vi "SyncMatrixGen (SubVI).vi"(9 "M":i32, 10 "Hamming distance":i32, 11 "Length":i32) -> (3 "Array":i32[][](array[numeric]))   [LabVIEW 2017]
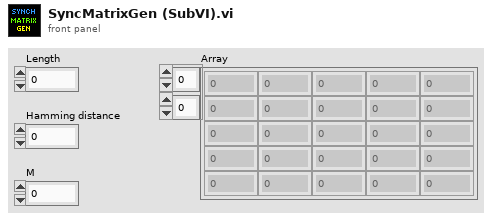
[diagram p1: front panel]
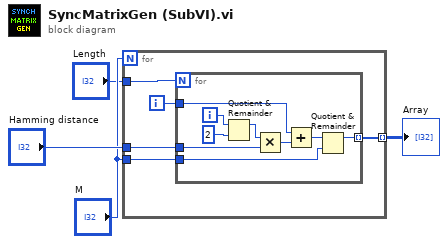
[diagram p0: block diagram]
diagram:
  n1 = for {
    N: "M" -> [_]
    tunnel: "Length" -> [w9]
    tunnel: [w8] -> w2 mode=indexing
    tunnel: "M" -> [w6]
    tunnel: "Hamming distance" -> [w5]
    i -> [w7]
    n2 = for {
      N: w9 -> [_]
      tunnel: [w12] -> w8 mode=indexing
      tunnel: w7 -> [w14]
      tunnel: w6 -> [w11]
      tunnel: w5 -> [w10]
      i -> [w18]
      n3 = Quotient & Remainder(x=w18, y=2) -> (x-y*floor(x/y)=w16:i32)  [unwired: 1 out]
      n4 = Multiply(x=w16, y=w10) -> (x*y=w15:i32)
      n5 = Add(x=w14, y=w15) -> (x+y=w13:i32)
      n6 = Quotient & Remainder(x=w13, y=w11) -> (x-y*floor(x/y)=w12:i32)  [unwired: 1 out]
    }
  }
  "Array" <- w2
